vi "Configure Channel.vi"(0 "VISA resource name":refnum<visa-resource-name>, 1 "Enable Channel (T:Enable)":bool=TRUE, 5 "Channel (1: Channel 1)":u16(ring)=1 items=["Channel 1"=1, "Channel 2"=2, "Channel 3"=3, "Channel 4"=4], 7 "Vertical Coupling (0: DC)":u16(ring) items=["DC", "AC", "Ground"], 9 "Probe Attenuation (1.0)":dbl=1.0, 11 "error in (no error)":errorcluster, 12 "Vertical Range (1.0 V)":dbl=1.0, 13 "Vertical Offset (0.0 V)":dbl) -> (4 "VISA resource name out":refnum<visa-resource-name>, 15 "error out":errorcluster)   [LabVIEW 2015, in "RIGOL DS1000 Series.lvlib"]
doc: "Configures the common properties of the vertical subsystem of the oscilloscope for the specified channel."
uses:
  RIGOL DS1000 Series.lvlib
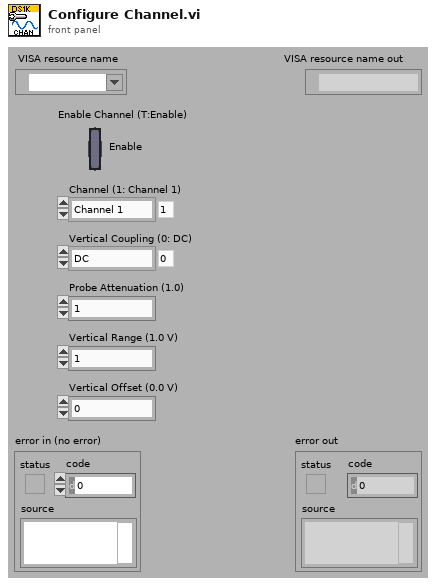
[diagram p1: front panel]
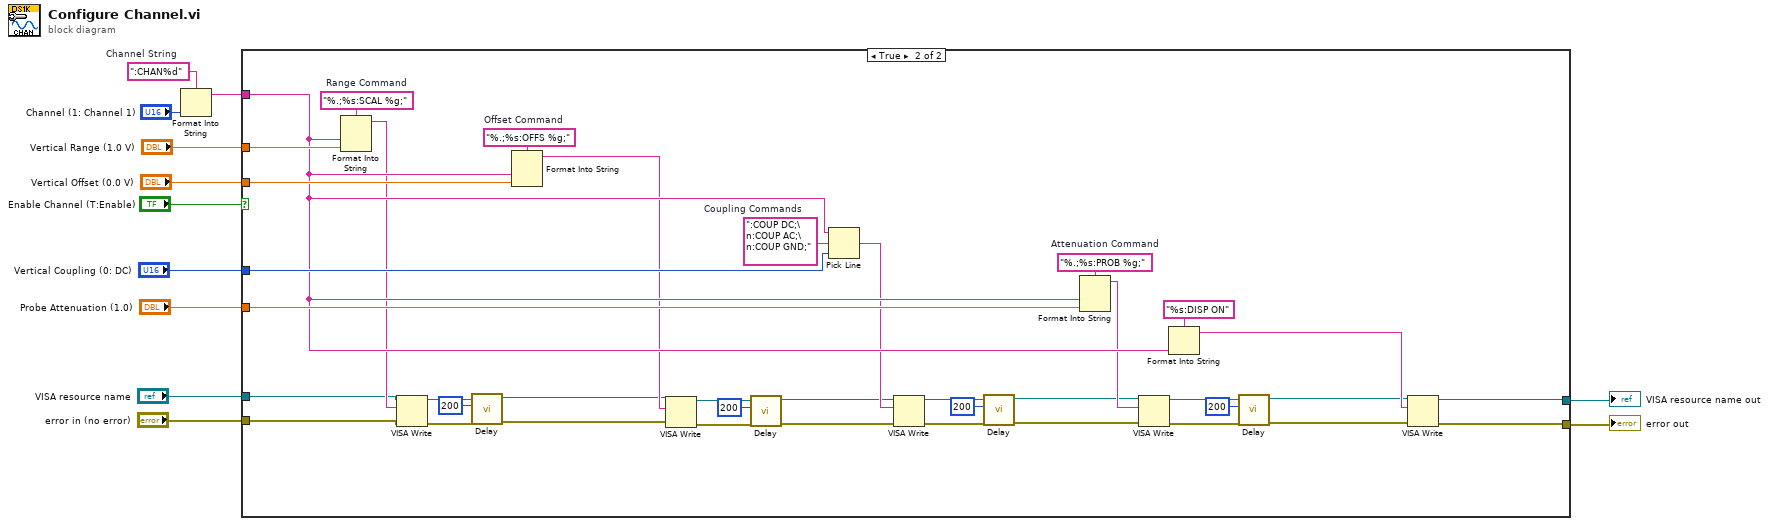
[diagram p0: block diagram]
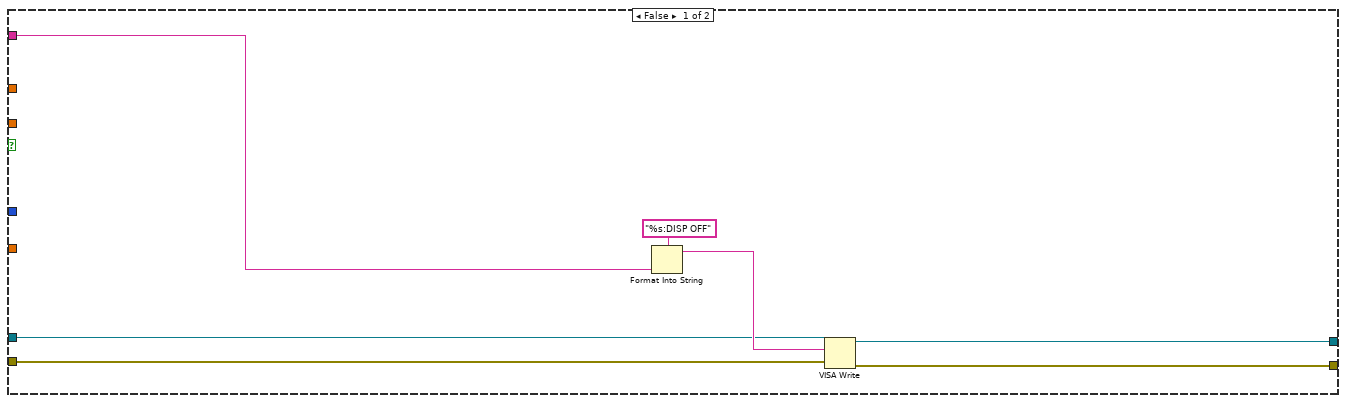
[diagram p2: hidden frame]
diagram:
  w10 = ":CHAN%d"  # Channel String
  n1 = Format Into String(format string=w10, "Channel (1: Channel 1)") -> (resulting string=w9:string)  [unwired: 2 in, 1 out]
  n2 = case shown="True" "Enable Channel (T:Enable)" {
    tunnel: w9 -> [w18 w49]
    tunnel: "Vertical Range (1.0 V)" -> [_ w53]
    tunnel: "Vertical Offset (0.0 V)" -> [_ w52]
    tunnel: "Vertical Coupling (0: DC)" -> [_ w51]
    tunnel: "Probe Attenuation (1.0)" -> [_ w50]
    tunnel: [w13 w20] -> w3
    tunnel: [w14 w21] -> w4
    tunnel: "VISA resource name" -> [w16 w43]
    tunnel: "error in (no error)" -> [w15 w42]
    frame False {
      n3 = Format Into String(format string="%s:DISP OFF", w18) -> (resulting string=w17:string)  [unwired: 2 in, 1 out]
      n4 = VISA Write(VISA resource name=w16, write buffer=w17, error in (no error)=w15) -> (VISA resource name out=w14:refnum<visa-resource-name>, error out=w13:errorcluster)  [unwired: 1 out]
    }
    frame True {
      w55 = "%.;%s:PROB %g;"  # Attenuation Command
      w56 = "%.;%s:SCAL %g;"  # Range Command
      w57 = "%.;%s:OFFS %g;"  # Offset Command
      w58 = ":COUP DC;\n:COUP AC;\n:COUP GND;"  # Coupling Commands
      n5 = Format Into String(format string=w56, w49, w53) -> (resulting string=w48:string)  [unwired: 2 in, 1 out]
      n6 = VISA Write(VISA resource name=w43, write buffer=w48, error in (no error)=w42) -> (VISA resource name out=w41:refnum<visa-resource-name>, error out=w40:errorcluster)  [unwired: 1 out]
      n7 = call "Delay.vi"("error in (no error)"=w40, "Delay (ms)"=u32 200, "VISA resource name"=w41) -> ("error out"=w28:errorcluster, "VISA resource name out"=w29:refnum<visa-resource-name>)  [unwired: 7 out]
      n8 = Format Into String(format string=w57, w49, w52) -> (resulting string=w47:string)  [unwired: 2 in, 1 out]
      n9 = VISA Write(VISA resource name=w29, write buffer=w47, error in (no error)=w28) -> (VISA resource name out=w39:refnum<visa-resource-name>, error out=w38:errorcluster)  [unwired: 1 out]
      n10 = call "Delay.vi"("error in (no error)"=w38, "Delay (ms)"=u32 200, "VISA resource name"=w39) -> ("error out"=w26:errorcluster, "VISA resource name out"=w27:refnum<visa-resource-name>)  [unwired: 7 out]
      n11 = Pick Line(string ("")=w49, multi-line string=w58, line index=w51) -> (output string=w46:string)
      n12 = VISA Write(VISA resource name=w27, write buffer=w46, error in (no error)=w26) -> (VISA resource name out=w37:refnum<visa-resource-name>, error out=w36:errorcluster)  [unwired: 1 out]
      n13 = call "Delay.vi"("error in (no error)"=w36, "Delay (ms)"=u32 200, "VISA resource name"=w37) -> ("error out"=w24:errorcluster, "VISA resource name out"=w25:refnum<visa-resource-name>)  [unwired: 7 out]
      n14 = Format Into String(format string=w55, w49, w50) -> (resulting string=w45:string)  [unwired: 2 in, 1 out]
      n15 = VISA Write(VISA resource name=w25, write buffer=w45, error in (no error)=w24) -> (VISA resource name out=w35:refnum<visa-resource-name>, error out=w34:errorcluster)  [unwired: 1 out]
      n16 = Format Into String(format string="%s:DISP ON", w49) -> (resulting string=w44:string)  [unwired: 2 in, 1 out]
      n17 = call "Delay.vi"("error in (no error)"=w34, "Delay (ms)"=u32 200, "VISA resource name"=w35) -> ("error out"=w22:errorcluster, "VISA resource name out"=w23:refnum<visa-resource-name>)  [unwired: 7 out]
      n18 = VISA Write(VISA resource name=w23, write buffer=w44, error in (no error)=w22) -> (VISA resource name out=w21:refnum<visa-resource-name>, error out=w20:errorcluster)  [unwired: 1 out]
    }
  }
  "error out" <- w3
  "VISA resource name out" <- w4
